vi "Actor Core.vi"(8 "error in":errorcluster, 11 "Countdown Timer in":refnum<class "Countdown Timer.lvclass">) -> (0 "error out":errorcluster, 3 "Actor out":refnum<class "Actor.lvclass">)   [LabVIEW 2015, in "Countdown Timer.lvlib" / "Countdown Timer.lvclass"]
doc: "(<B>Filename</B>: Actor Framework.lvlib:Actor.lvclass:Actor Core.vi)\n\nReceives messages to the actor, reacts to them, and initiates any error handling that may shut the actor down.\n\nDescendant classes may override this VI to append parallel tasks for the actor to complete while it handles messages. Overrides use the Call Parent Method node."
uses:
  Countdown Timer.lvclass
  UI Window/UI Window.lvclass
  <vilib>/ActorFramework/Actor/Actor.lvclass
  <vilib>/ActorFramework/Stop Msg/Stop Msg.lvclass
  Resources/GLOBAL/GLOBAL Time-critical.vi
panel:
  out "Countdown Message":string
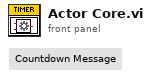
[diagram p1: front panel]
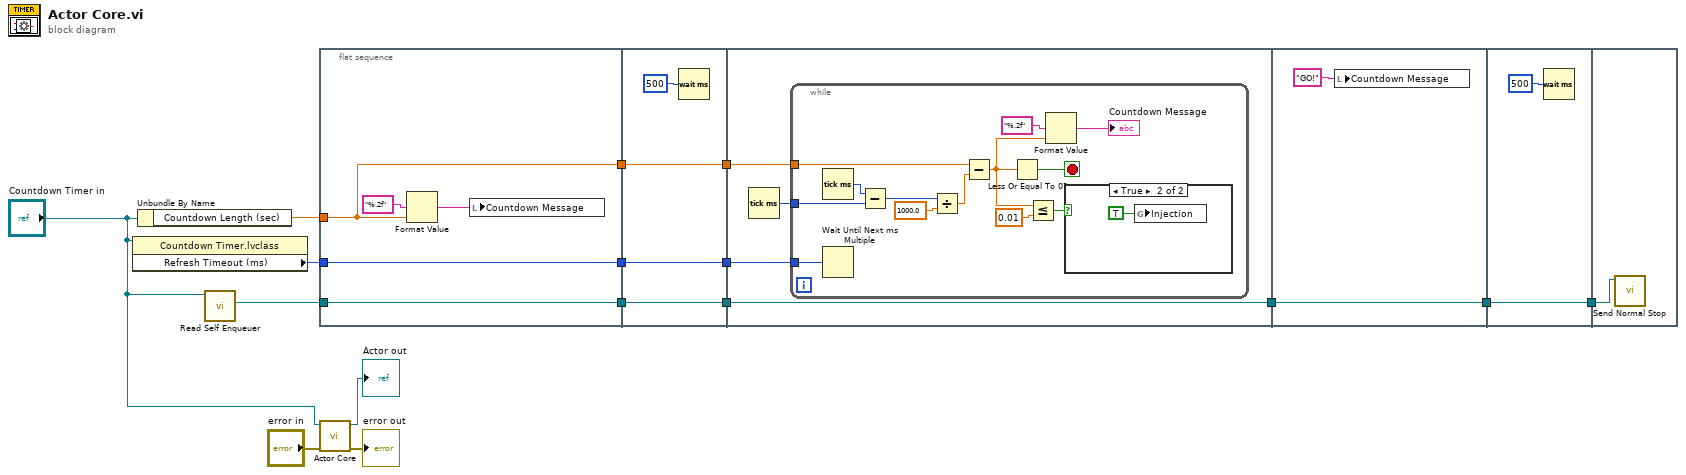
[diagram p0: block diagram]
diagram:
  n1 = property class="Countdown Timer.lvclass"(reference="Countdown Timer in") -> ("Refresh Timeout (ms)"=w6:i32)  [unwired: 1 in, 2 out]
  n2 = Unbundle By Name("Countdown Timer in") -> ("Countdown Length (sec)"=w4:dbl)
  n3 = call <vilib>:"Read Self Enqueuer.vi"("Actor"="Countdown Timer in") -> ("Self Enqueuer"=w13:refnum<class "Message Enqueuer.lvclass">)  [unwired: 10 in]
  n4 = flat-sequence {
    tunnel: w6 -> [w20]
    tunnel: w13 -> [w21]
    tunnel: w4 -> [w17]
    tunnel: [w17] -> w3
    tunnel: [w21] -> w2
    tunnel: [w20] -> w1
    tunnel: [w25] -> w11
    tunnel: [w24] -> w10
    tunnel: [w22] -> w5
    tunnel: w3 -> [w25]
    tunnel: w2 -> [w24]
    tunnel: w1 -> [w22]
    tunnel: [w27] -> w12
    tunnel: w11 -> [w28]
    tunnel: w10 -> [w27]
    tunnel: w5 -> [w26]
    tunnel: w12 -> [w44]
    tunnel: [w44] -> w8
    tunnel: [w46] -> w9
    tunnel: w8 -> [w46]
    tunnel: w9 -> [w48]
    frame #0 {
      n5 = Format Value(format string="%.2f", value (0)=w17) -> (output string=w19:string)  [unwired: 1 in]
      n6 = local write "Countdown Message"(w19) -> ()
    }
    frame #1 {
      n7 = Wait (ms)(milliseconds to wait=u32 500) -> ()  [unwired: 1 out]
    }
    frame #2 {
      n8 = Tick Count (ms)() -> (millisecond timer value=w29:u32)
      n9 = while {
        tunnel: w29 -> [w40]
        tunnel: w28 -> [w36]
        tunnel: w26 -> [w33]
        stop <- w42 stop-if-true
        n10 = Tick Count (ms)() -> (millisecond timer value=w41:u32)
        n11 = Wait Until Next ms Multiple(millisecond multiple=w33) -> ()  [unwired: 1 out]
        n12 = Subtract(x=w41, y=w40) -> (x-y=w39:u32)
        n13 = Divide(x=w39, y=1000.0) -> (x/y=w37:dbl)
        n14 = Subtract(x=w36, y=w37) -> (x-y=w32:dbl)
        n15 = Less Or Equal To 0?(x=w32) -> (x <= 0?=w42:bool)
        n16 = Less Or Equal?(x=w32, y=0.01) -> (x <= y?=w30:bool)
        n17 = Format Value(format string="%.2f", value (0)=w32) -> (output string=→"Countdown Message":string)  [unwired: 1 in]
        n18 = case shown="True" w30 {
          frame False {
          }
          frame True {
            n19 = global write "GLOBAL Time-critical.vi" "Injection"(TRUE ("Injection")) -> ()
          }
        }
      }
    }
    frame #3 {
      n20 = local write "Countdown Message"("GO!" ("Countdown Message")) -> ()
    }
    frame #4 {
      n21 = Wait (ms)(milliseconds to wait=u32 500) -> ()  [unwired: 1 out]
    }
    frame #5 {
      n22 = call <vilib>:"Send Normal Stop.vi"("Message Enqueuer"=w48) -> ()  [unwired: 10 in, 1 out]
    }
  }
  n23 = call-parent "Actor Core.vi"("error in"="error in", "UI Window in"="Countdown Timer in") -> ("error out"=→"error out":errorcluster, "Actor out"=→"Actor out":refnum<class "Actor.lvclass">)  [unwired: 8 in]
